vi "SwissSPAD Live_Init Communication v2.vi"(8 "Error In":errorcluster, 11 "SwissSPAD Live Internal Variables in":T2={"okCFrontPanelDevices Refnum"=refnum, "Bottom Device Refnum"=refnum, "Display Image"=refnum, "# Live Images"=0, "relative s"=0.0, "# Image Sets"=0, "Message"="", "Current Image Set"=0, "# Datasets in Series"=0, "Current Dataset"=0, "Live Mode"=FALSE, "Recording Mode"=FALSE, "Record Button"=refnum, "\nLive Button"=refnum, "SwissSPAD Live Gate Image Data Q Name"="SS2 Live Gate Data Q", "Discard First Image"=FALSE, "Image Information"={"Save ROI Only"=FALSE, "Left"=0, "Top"=0, "Right"=0, "Bottom"=0, "Use Current ROI"=FALSE}, "Image Binning Options"={"Use Image Binning"=FALSE, "X Bin"=1, "Y Bin"=1}, "Bottom FPGA Serial Number"="", "Detector PCB Version"=enum."SS2 PCB1", "# Acquisitions"=1, "10 bits"=FALSE, "Top FPGA Serial Number"="", "Top Device Refnum"=refnum} {"# Acquisitions" min=1; "Image Binning Options"."Y Bin" min=1; "Image Binning Options"."X Bin" min=1}) -> (0 "Error Out":errorcluster, 1 "Init Communication Outcome":T1, 3 "SwissSPAD Live Internal Variables out":T2={"okCFrontPanelDevices Refnum"=refnum, "Bottom Device Refnum"=refnum, "Display Image"=refnum, "# Live Images"=0, "relative s"=0.0, "# Image Sets"=0, "Message"="", "Current Image Set"=0, "# Datasets in Series"=0, "Current Dataset"=0, "Live Mode"=FALSE, "Recording Mode"=FALSE, "Record Button"=refnum, "\nLive Button"=refnum, "SwissSPAD Live Gate Image Data Q Name"="SS2 Live Gate Data Q", "Discard First Image"=FALSE, "Image Information"={"Save ROI Only"=FALSE, "Left"=0, "Top"=0, "Right"=0, "Bottom"=0, "Use Current ROI"=FALSE}, "Image Binning Options"={"Use Image Binning"=FALSE, "X Bin"=1, "Y Bin"=1}, "Bottom FPGA Serial Number"="", "Detector PCB Version"=enum."SS2 PCB1", "# Acquisitions"=1, "10 bits"=FALSE, "Top FPGA Serial Number"="", "Top Device Refnum"=refnum} {"# Acquisitions" min=1; "Image Binning Options"."Y Bin" min=1; "Image Binning Options"."X Bin" min=1})   [LabVIEW 2021]
uses:
  SwissSPAD Live_Internal Variables.ctl
  D:/UCLA Thinkpad Google Drive/LabVIEW 2021 SP1/builds/SwissSPAD Live Distribution/Opal Kelly/C# Wrapper/v5.0.2/libFrontPanel-csharp.dll
  Opal Kelly/C# Wrapper/v5.0.2/libFrontPanel-csharp.dll
  <vilib>/vision/Image Controls.llb/IMAQ Image.ctl
  SwissSPAD Live_Image ROI Information.ctl
  Phasor/Image Binning Options.ctl
  SwissSPAD Live_SSx PCB Version.ctl
  SwissSPAD Live_Init Communication Outcome.ctl
  SwissSPAD Live_Internal Data List.ctl
  Opal Kelly/C# Wrapper/okFrontPanelC#Wrapper.lvlib
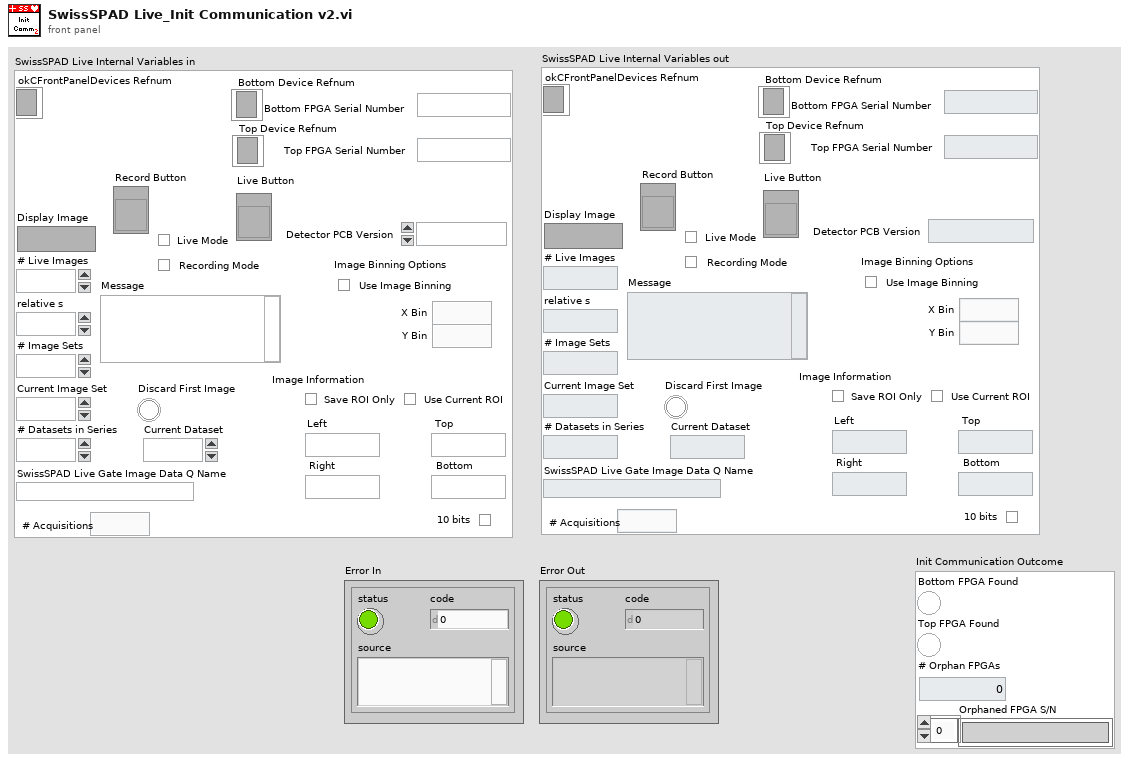
[diagram p1: front panel]
types:
  T1 = typedef "SwissSPAD Live_Init Communication Outcome.ctl" = cluster{"Bottom FPGA Found":bool, "Top FPGA Found":bool, "# Orphan FPGAs":i32, "Orphaned FPGA S/N":string[]}
  T2 = typedef "SwissSPAD Live_Internal Variables.ctl" = cluster{"okCFrontPanelDevices Refnum":refnum<k24>, "Bottom Device Refnum":refnum<k24>, "Display Image":T3, "# Live Images":i32, "relative s":dbl, "# Image Sets":i32, "Message":string, "Current Image Set":i32, "# Datasets in Series":i32, "Current Dataset":i32, "Live Mode":bool, "Recording Mode":bool, "Record Button":refnum<vi>, "\nLive Button":refnum<vi>, "SwissSPAD Live Gate Image Data Q Name":string, "Discard First Image":bool, "Image Information":T4, "Image Binning Options":T5, "Bottom FPGA Serial Number":string, "Detector PCB Version":T6, "# Acquisitions":u32, "10 bits":bool, "Top FPGA Serial Number":string, "Top Device Refnum":refnum<k24>}
  T3 = typedef "IMAQ Image.ctl" = refnum<image>
  T4 = typedef "SwissSPAD Live_Image ROI Information.ctl" = cluster{"Save ROI Only":bool, "Left":u16, "Top":u16, "Right":u16, "Bottom":u16, "Use Current ROI":bool}
  T5 = typedef "Image Binning Options.ctl" = cluster{"Use Image Binning":bool, "X Bin":i32, "Y Bin":i32}
  T6 = typedef "SwissSPAD Live_SSx PCB Version.ctl" = enum16{"unknown", "SS2 PCB1", "SS2 PCB2", "SS3 PCB1"}
  T7 = typedef "SwissSPAD Live_Internal Data List.ctl" = enum16{"Number of pending file saving tasks", "File Saving Tasks Information", "Current Image ROI Information", "# FPGA Reset Attempts", "Histogram Cursor Locations", "Histogram Window is Open"}
  T8 = typedef "okFrontPanelC#Wrapper.lvlib/okTDeviceInfo Struct.ctl" = cluster{"deviceID":string, "okInterface":T9, "deviceMajorVersion":i32, "deviceMinorVersion":i32, "FPGA Flash Memory Layout":T10, "System Flash Memory Layout":T10, "hasFMCEEPROM":bool, "hasResetProfiles":bool, "hostInterfaceMajorVersion":i32, "hostInterfaceMinorVersion":i32, "isFrontPanelEnabled":bool, "isPLL22150Supported":bool, "isPLL22393Supported":bool, "pipeWidth":i32, "Device ID":T11, "productName":string, "registerAddressWidth":i32, "registerDataWidth":i32, "serialNumber":string, "triggerWidth":i32, "USB Speed":T12, "wireWidth":i32}
  T9 = typedef "okFrontPanelC#Wrapper.lvlib/okEDeviceInterface.ctl" = enum16{"unknown", "USB2", "PCIe", "USB3"}
  T10 = typedef "okFrontPanelC#Wrapper.lvlib/okTFlashLayoutStruct.ctl" = cluster{"maxUserSector":u32, "minUserSector":u32, "pageSize":u32, "sectorCount":u32, "sectorSize":u32}
  T11 = typedef "okFrontPanelC#Wrapper.lvlib/okTProductID.ctl" = enum16{"UNKNOWN", "XEM3001V1", "XEM3001V2", "XEM3010", "XEM3005", "XEM3001CL", "XEM3020", "XEM3050", "XEM9002", "XEM3001RB", "XEM5010", "XEM6110LX45", "XEM6001", "XEM6010LX45", "XEM6010LX150", "XEM6110LX150", "XEM6006LX9", "XEM6006LX16", "XEM6006LX25", "XEM5010LX110", "ZEM4310", "XEM6310LX45", "XEM6310LX150", "XEM6110V2LX45", "XEM6110V2LX150", "XEM6002LX9", "XEM6310MTLX45T", "XEM6320LX130T", "XEM7350K70T", "XEM7350K160T", "XEM7350K410T", "XEM6310MTLX150T", "ZEM5305A2", "ZEM5305A7", "XEM7001A15", "XEM7001A35", "XEM7360K160T", "XEM7360K410T", "ZEM5310A4", "ZEM5310A7", "ZEM5370A5", "XEM7010A50", "XEM7010A200", "XEM7310A75", "XEM7310A200", "XEM7320A75T", "XEM7320A200T", "XEM7305", "FPXBARE"}
  T12 = typedef "okFrontPanelC#Wrapper.lvlib/okEUSBSpeed.ctl" = enum16{"unknown", "Full", "High", "Super"}
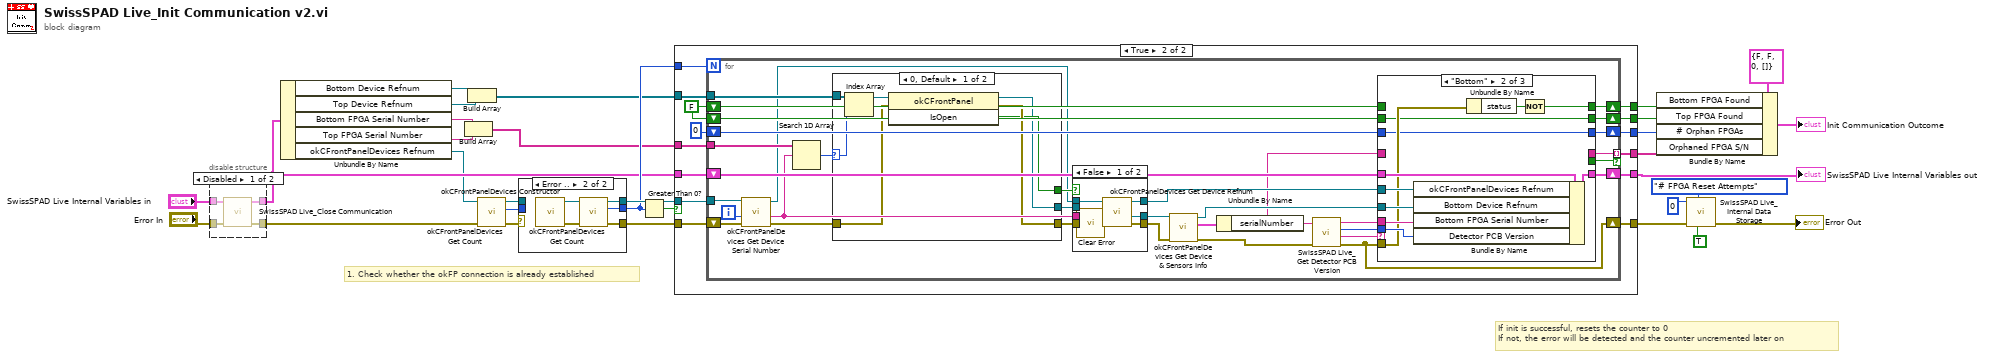
[diagram p0: block diagram]
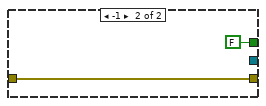
[diagram p4: hidden frame]
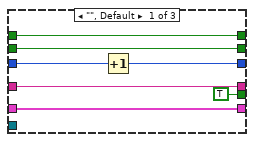
[diagram p5: hidden frame]
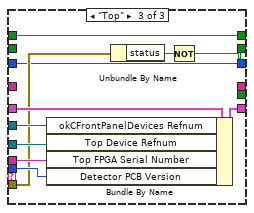
[diagram p6: hidden frame]
diagram:
  # "1. Check whether the okFP connection is already established"
  # "If init is successful, resets the counter to 0\nIf not, the error will be detected and the counter uncremented later on"
  n1 = disable-structure shown="Disabled" {
    disable-tunnel: "Error In" -> [w34 w35]
    disable-tunnel: [w33 w35] -> w10
    disable-tunnel: "SwissSPAD Live Internal Variables in" -> [w32 w36]
    disable-tunnel: [w31 w36] -> w12
    frame Disabled {
      n2 = call "SwissSPAD Live_Close Communication.vi"("Error In"=w34, "SwissSPAD Live Internal Variables"=w32) -> ("Error Out"=w33:errorcluster, "SwissSPAD Live Internal Variables"=w31:T2)  [unwired: 8 in]
    }
    frame Enabled {
    }
  }
  n3 = Unbundle By Name(w12) -> ("Bottom Device Refnum"=w3:refnum<k24>, "Top Device Refnum"=w2:refnum<k24>, "Bottom FPGA Serial Number"=w6:string, "Top FPGA Serial Number"=w5:string, "okCFrontPanelDevices Refnum"=w11:refnum<k24>)
  n4 = Build Array(w6, w5) -> (w4:string[])
  n5 = Build Array(w3, w2) -> (w1:refnum<k24>[])
  n6 = call "okCFrontPanelDevices Get Count.vi"("Error In"=w10, "okCFrontPanelDevices Refnum"=w11) -> ("Error Out"=w9:errorcluster, "GetCount"=w8:i32, "okCFrontPanelDevices Refnum"=w7:refnum<k24>)  [unwired: 7 in]
  n7 = case shown="Error .." w9 {
    selector: w9 -> [w39 _]
    tunnel: [w37 w42] -> w30
    tunnel: [w39 w41] -> w28
    tunnel: [w38 w40] -> w15
    tunnel: w8 -> [w38 _]
    tunnel: w7 -> [w37 _]
    frame No Error {
    }
    frame Error {
      n8 = call "okCFrontPanelDevices Constructor.vi"() -> ("Error Out"=w44:errorcluster, "okCFrontPanelDevices Refnum"=w43:refnum<k24>)  [unwired: 10 in]
      n9 = call "okCFrontPanelDevices Get Count.vi"("Error In"=w44, "okCFrontPanelDevices Refnum"=w43) -> ("Error Out"=w41:errorcluster, "GetCount"=w40:i32, "okCFrontPanelDevices Refnum"=w42:refnum<k24>)  [unwired: 7 in]
    }
  }
  n10 = Greater Than 0?(x=w15) -> (x > 0?=w29:bool)
  n11 = case shown="True" w29 {
    tunnel: w30 -> [_ w60]
    tunnel: w28 -> [w46 w59]
    tunnel: [w46 w58] -> w23
    tunnel: w15 -> [_ w57]
    tunnel: w12 -> [w45 w56]
    tunnel: [w45 w55] -> w22
    tunnel: [_ w53] -> w21
    tunnel: [_ w52] -> w20
    tunnel: [_ w50] -> w19
    tunnel: [_ w49] -> w18
    tunnel: w4 -> [_ w48]
    tunnel: w1 -> [_ w47]
    frame False {
    }
    frame True {
      w54 = FALSE ("Bottom FPGA Reset")
      n12 = for {
        N: w57 -> [_]
        shift-right: [w80] -> w58
        shift-left: w59 -> [w92]
        shift-right: [w83] -> w55
        shift-left: w56 -> [w86]
        tunnel: w60 -> [w93]
        shift-right: [w76] -> w53
        shift-left: w54 -> [w77]
        shift-right: [w78] -> w52
        shift-left: w54 -> [w79]
        shift-right: [w74] -> w50
        shift-left: 0 -> [w75]
        tunnel: [w72] -> w49 mode=indexing if=w71
        tunnel: w48 -> [w69]
        tunnel: w47 -> [w66]
        i -> [w88]
        n13 = call "okCFrontPanelDevices Get Device Serial Number.vi"("Error In"=w92, "Device ID"=w88, "okCFrontPanelDevices Refnum"=w93) -> ("Error Out"=w65:errorcluster, "Serial Number"=w68:string, "okCFrontPanelDevices Refnum"=w61:refnum<k24>)  [unwired: 6 in]
        n14 = Search 1D Array(1D array=w69, element=w68) -> (index of element=w67:i32)  [unwired: 1 in]
        n15 = case shown="0, Default" w67 {
          selector: w67 -> [w109 _]
          tunnel: w66 -> [w110 _]
          tunnel: w65 -> [w107 w112]
          tunnel: [w106 w112] -> w64
          tunnel: [w105 FALSE ("IsOpen")] -> w63
          tunnel: [w104 _] -> w62
          frame 0, Default {
            n16 = Index Array(array=w110, index=w109) -> (element=w108:refnum<k24>)
            n17 = invoke class="okCFrontPanel" method="IsOpen"(reference=w108, error in=w107) -> (reference out=w104:refnum<k24>, error out=w106:errorcluster, "IsOpen"=w105:bool)  [unwired: 1 in]
          }
          frame -1 {
          }
        }
        n18 = case shown="False" w63 {
          tunnel: [w100 w102] -> w91
          tunnel: w61 -> [w99 w103]
          tunnel: [w98 w103] -> w82
          tunnel: [w97 w101] -> w70
          tunnel: w68 -> [w96 _]
          tunnel: w64 -> [w95 w102]
          tunnel: w62 -> [_ w101]
          frame False {
            n19 = call "Clear Error.vi"("Error In"=w95) -> ("no Error Out"=w94:errorcluster)  [unwired: 8 in]
            n20 = call "okCFrontPanelDevices Get Device Refnum.vi"("Error In"=w94, "Serial Number"=w96, "okCFrontPanelDevices Refnum"=w99) -> ("Error Out"=w100:errorcluster, "Device Refnum"=w97:refnum<k24>, "okCFrontPanelDevices Refnum"=w98:refnum<k24>)  [unwired: 6 in]
          }
          frame True {
          }
        }
        n21 = call "okCFrontPanelDevices Get Device & Sensors Info.vi"("error in (no error)"=w91, "okCFrontPanel Device Refnum"=w70) -> ("error out"=w89:errorcluster, "Device Info"=w90:T8, "okCFrontPanel Device Refnum"=w85:refnum<k24>)  [unwired: 5 in, 2 out]
        n22 = Unbundle By Name(w90) -> ("serialNumber"=w73:string)
        n23 = call "SwissSPAD Live_Get Detector PCB Version.vi"("error in (no error)"=w89, "serialNumber"=w73) -> ("error out"=w80:errorcluster, "Sensor Part"=w87:string, "PCB Version"=w81:T6, "serialNumber (dup)"=w84:string)  [unwired: 6 in]
        n24 = case shown="\"Bottom\"" w87 {
          tunnel: w86 -> [w119 w130 w141]
          tunnel: w85 -> [_ w128 w139]
          tunnel: w84 -> [_ w129 w140]
          tunnel: [w119 w127 w138] -> w83
          tunnel: w82 -> [_ w126 w137]
          tunnel: w81 -> [_ w125 w136]
          tunnel: [w118 w122 w135] -> w76
          tunnel: w80 -> [_ w124 w133]
          tunnel: w79 -> [w117 w121 _]
          tunnel: [w117 w121 w132] -> w78
          tunnel: w77 -> [w118 _ w135]
          tunnel: w75 -> [w116 w120 w131]
          tunnel: [w115 w120 w131] -> w74
          tunnel: [w114 _ _] -> w72
          tunnel: w73 -> [w114 _ _]
          tunnel: [TRUE _ _] -> w71
          frame "", Default {
            n25 = Increment(x=w116) -> (x+1=w115:i32)
          }
          frame "Bottom" {
            n26 = Bundle By Name(cluster=w130, "okCFrontPanelDevices Refnum"=w126, "Bottom Device Refnum"=w128, "Bottom FPGA Serial Number"=w129, "Detector PCB Version"=w125) -> (w127:T2)
            n27 = Unbundle By Name(w124) -> ("status"=w123:bool)
            n28 = Not(x=w123) -> (.not. x?=w122:bool)
          }
          frame "Top" {
            n29 = Bundle By Name(cluster=w141, "okCFrontPanelDevices Refnum"=w137, "Top Device Refnum"=w139, "Top FPGA Serial Number"=w140, "Detector PCB Version"=w136) -> (w138:T2)
            n30 = Unbundle By Name(w133) -> ("status"=w134:bool)
            n31 = Not(x=w134) -> (.not. x?=w132:bool)
          }
        }
      }
    }
  }
  "SwissSPAD Live Internal Variables out" <- w22
  n32 = Bundle By Name(cluster=T1 {"Bottom FPGA Found"=FALSE, "Top FPGA Found"=FALSE, "# Orphan FPGAs"=0, "Orphaned FPGA S/N"=[]} ("Init Communication Outcome"), "Bottom FPGA Found"=w21, "Top FPGA Found"=w20, "# Orphan FPGAs"=w19, "Orphaned FPGA S/N"=w18) -> (→"Init Communication Outcome":T1)
  n33 = call "SwissSPAD Live_Internal Data Storage.vi"("Get(F)/Set"=TRUE, "SS2 Live Data"=SwissSPAD_Live_Internal_Data_List."# FPGA Reset Attempts", "Error In"=w23, "Variant"=0 ("y")) -> ("Error Out"=→"Error Out":errorcluster)  [unwired: 5 in, 2 out]
